vi "Receive messege by module.vi"(8 "error in (no error)":errorcluster, 9 "timeout in ms (-1)":i32=-1, 11 "Module mailbox":T1) -> (0 "error out":errorcluster, 2 "Unread":i32, 3 "Data":variant, 4 "timed out?":bool, 5 "queue name":string)   [LabVIEW 2018, in "MessengerLib.lvlib"]
uses:
  MessengerLib.lvlib
  Data types/Mailbox address.ctl
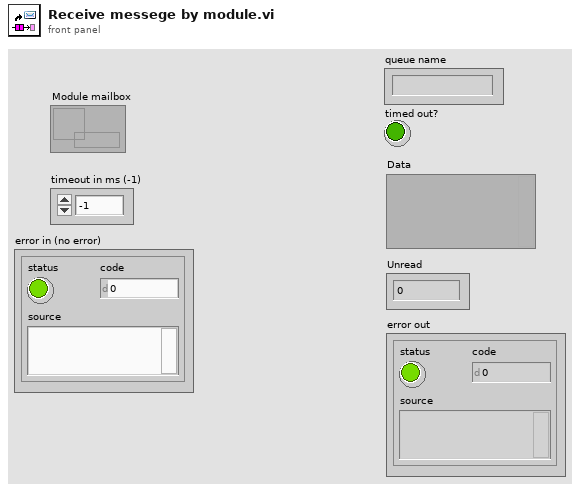
[diagram p1: front panel]
types:
  T1 = typedef "MessengerLib.lvlib/Mailbox address.ctl" = refnum<queue>
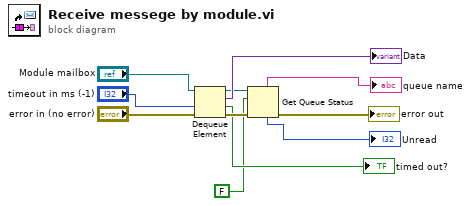
[diagram p0: block diagram]
diagram:
  n1 = Dequeue Element(queue="Module mailbox", timeout in ms (-1)="timeout in ms (-1)", error in (no error)="error in (no error)") -> (queue out=w8:T1, element=→"Data":variant, timed out?=→"timed out?":bool, error out=w7:errorcluster)
  n2 = Get Queue Status(queue=w8, return elements? (F)=FALSE, error in (no error)=w7) -> (queue name=→"queue name":string, error out=→"error out":errorcluster, # elements in queue=→"Unread":i32)  [unwired: 5 out]
